vi "EEISysLink Test Harness subVI.vi"(8 "error in (no error)":errorcluster, 11 "EEISysLink in":refnum<class "EEISysLink.lvclass">) -> (0 "error out":errorcluster, 1 "Tag Server Updates":i32, 2 "Tag Values 2":T1[](array[typedef]), 3 "EEISysLink out":refnum<class "EEISysLink.lvclass">)   [LabVIEW 2016]
uses:
  Controls/SL Tag Value.ctl
  Controls/SL Tag Data Type.ctl
  EEISysLink.lvclass
  Controls/SL Tag Scope.ctl
  Controls/SL Tag Type.ctl
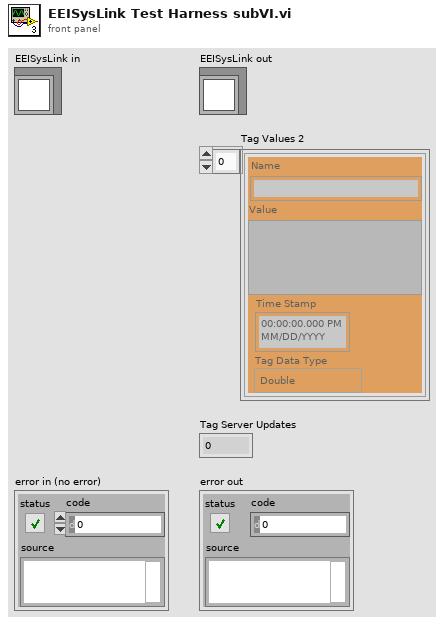
[diagram p1: front panel]
types:
  T1 = typedef "SL Tag Value.ctl" = cluster{"Value":variant, "Time Stamp":timestamp, "Tag Data Type":T2, "Name":string}
  T2 = typedef "EEISysLink.lvclass/SL Tag Data Type.ctl" = enum16{"Double", "Integer", "String", "Boolean", "Waveform"}
  T3 = typedef "EEISysLink.lvclass/SL Tag Type.ctl" = enum16{"All", "Supervisor", "Worker"}
  T4 = typedef "EEISysLink.lvclass/SL Tag Scope.ctl" = enum16{"Local", "Server"}
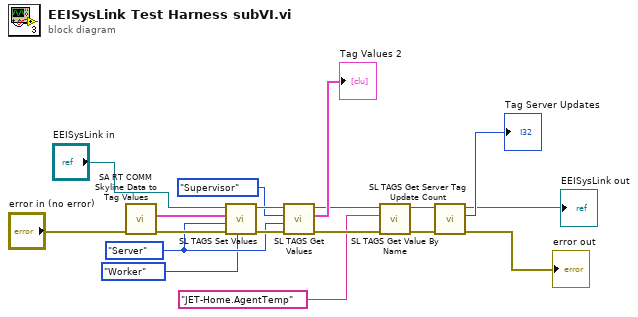
[diagram p0: block diagram]
diagram:
  w8 = SL_Tag_Scope."Server" ("Tag Scope")
  n1 = call "SA RT COMM Skyline Data to Tag Values.vi"("error in (no error)"="error in (no error)") -> ("error out"=w17:errorcluster, "Tag Values"=w15:T1[])  [unwired: 9 in]
  n2 = call-dynamic "SL TAGS Set Values.vi"("Tag Type"=SL_Tag_Type."Worker", "error in (no error)"=w17, "Tag Scope"=w8, "Tag Update Values"=w15, "EEISysLink in"="EEISysLink in") -> ("error out"=w11:errorcluster, "EEISysLink out"=w10:refnum<class "EEISysLink.lvclass">)  [unwired: 5 in]
  n3 = call-dynamic "SL TAGS Get Values.vi"("error in (no error)"=w11, "Tag Scope"=w8, "Tag Type"=SL_Tag_Type."Supervisor", "EEISysLink in"=w10) -> ("error out"=w4:errorcluster, "Tag Values"=→"Tag Values 2":T1[], "EEISysLink out"=w5:refnum<class "EEISysLink.lvclass">)  [unwired: 5 in]
  n4 = call-dynamic "SL TAGS Get Value By Name.vi"("error in (no error)"=w4, "Tag Name"="JET-Home.AgentTemp", "EEISysLink in"=w5) -> ("error out"=w2:errorcluster, "EEISysLink out"=w3:refnum<class "EEISysLink.lvclass">)  [unwired: 6 in, 1 out]
  n5 = call-dynamic "SL TAGS Get Server Tag Update Count.vi"("error in (no error)"=w2, "EEISysLink in"=w3) -> ("error out"=→"error out":errorcluster, "Tag Server Updates"=→"Tag Server Updates":i32, "EEISysLink out"=→"EEISysLink out":refnum<class "EEISysLink.lvclass">)  [unwired: 7 in]
